vi "Add_Props_Display.vi"(10 "Display":T1={"Alpha"=nan, "Z Order"=nan}, 11 "Keyword Array":T2[](array[typedef])) -> (3 "Keyword Array Out":T2[](array[typedef]))   [LabVIEW 2013, in "Advanced Plotting Toolkit.lvlib"]
uses:
  Advanced Plotting Toolkit.lvlib
  KeyValue.ctl
  properties/Display.ctl
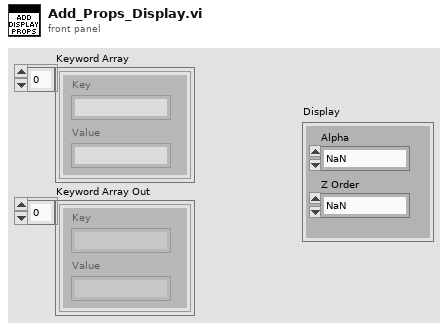
[diagram p1: front panel]
types:
  T1 = typedef "Advanced Plotting Toolkit.lvlib/Display.ctl" = cluster{"Alpha":dbl, "Z Order":dbl}
  T2 = typedef "Advanced Plotting Toolkit.lvlib/KeyValue.ctl" = cluster{"Key":string, "Value":string}
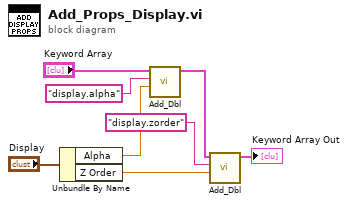
[diagram p0: block diagram]
diagram:
  n1 = Unbundle By Name("Display") -> ("Alpha"=w5:dbl, "Z Order"=w2:dbl)
  n2 = call "Add_Dbl.vi"("Value"=w5, "Key"="display.alpha", "Keyword Array"="Keyword Array") -> ("Keyword Array Out"=w4:T2[])  [unwired: 8 in]
  n3 = call "Add_Dbl.vi"("Value"=w2, "Key"="display.zorder", "Keyword Array"=w4) -> ("Keyword Array Out"=→"Keyword Array Out":T2[])  [unwired: 8 in]
